vi "run.vi"(8 "error in (no error)":errorcluster, 11 "GenericStimulator in":refnum<class "GenericStimulator.lvclass">) -> (0 "error out":errorcluster, 3 "GenericStimulator out":refnum<class "GenericStimulator.lvclass">)   [LabVIEW 2010, in "GenericStimulator.lvclass"]
uses:
  GenericStimulator.lvclass
panel:
  # "Functionality not available..."
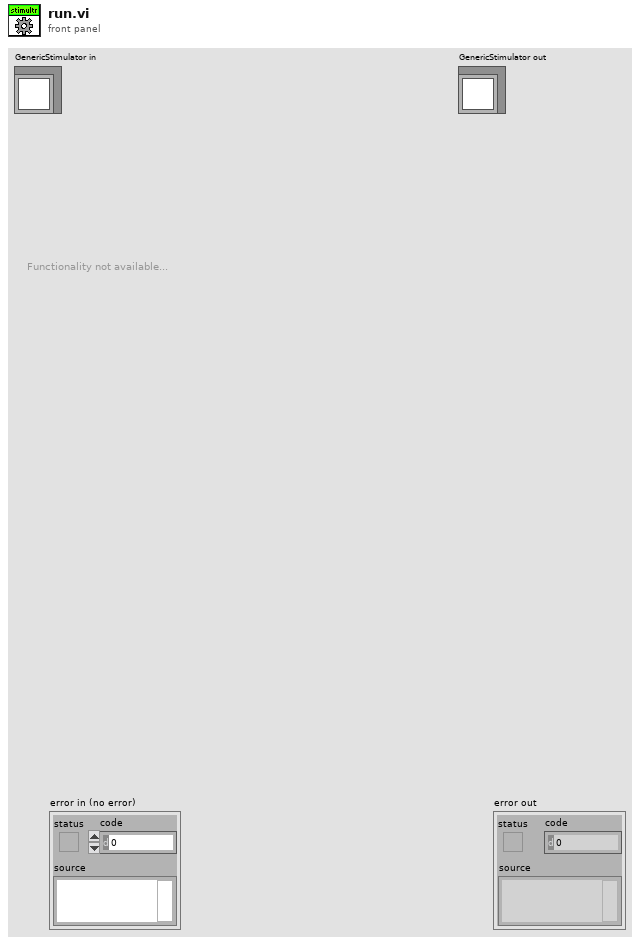
[diagram p1: front panel]
types:
  T1 = typedef "main_trigger_enum.ctl" = enum16{"NULL", "initialise", "terminate", "start", "stop", "change objective", "change experimentController", "change imagingMode", "save notebook", "started saving", "finished saving", "expCtr ready", "expCtr missing", "imgMd ready", "imgMd missing", "scanHd ready", "scanHd missing", "DAQ ready", "DAQ missing", "imgAsm ready", "imgAsm missing", "dataColl ready", "dataColl missing", "display ready", "display missing", "analysr ready", "analysr missing", "instrmnt ready", "instrmnt missing", "stimltr ready", "stimltr missing", "stage ready", "stage missing"}
  T2 = typedef "GenericToplevelComponent.lvclass/common_trigger_enum.ctl" = enum16{"NULL", "initialise", "terminate", "fetch command", "fetch data", "attach observer", "register as observer", "detach observer", "acknowledge", "start", "stop", "sweep started", "sweep finished", "experiment started", "experiment stopped"}
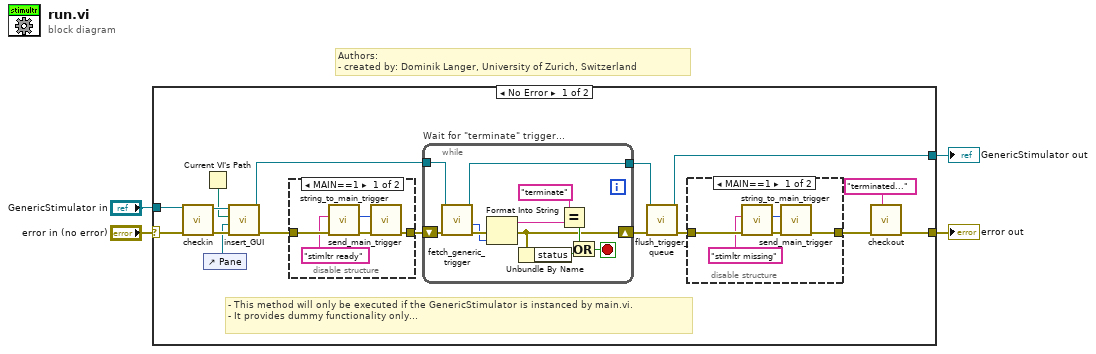
[diagram p0: block diagram]
diagram:
  # "Authors: \n- created by: Dominik Langer, University of Zurich, Switzerland"
  n1 = case shown="No Error" "error in (no error)" {
    selector: "error in (no error)" -> [w20 w45]
    tunnel: [w19 w45] -> w3
    tunnel: [w5 w44] -> w1
    tunnel: "GenericStimulator in" -> [w18 w44]
    frame No Error {
      # "- This method will only be executed if the GenericStimulator is instanced by main.vi.\n- It provides dummy functionality only..."
      n2 = call-dynamic "checkin.vi"("error in (no error)"=w20, "GenericStimulator in"=w18) -> ("error out"=w15:errorcluster, "GenericStimulator out"=w14:refnum<class "GenericStimulator.lvclass">)  [unwired: 8 in]
      n3 = Current VI's Path() -> (path=w13:path)
      n4 = control-ref of="Pane"() -> (w12:refnum<vi>)
      n5 = call-dynamic "insert_GUI.vi"("error in (no error)"=w15, "Pane"=w12, "VI path"=w13, "GenericComponent in"=w14) -> ("error out"=w11:errorcluster, "GenericComponent out"=w6:refnum<class "GenericStimulator.lvclass">)  [unwired: 6 in]
      n6 = disable-structure shown="MAIN==1" {
        disable-tunnel: w11 -> [w30 w32]
        disable-tunnel: [w31 w32] -> w16
        frame condition #0 (active) {
          n7 = call "string_to_main_trigger.vi"("error in (no error)"=w30, "trigger string"="stimltr ready") -> ("error out"=w29:errorcluster, "main trigger"=w28:T1)  [unwired: 8 in]
          n8 = call "send_main_trigger.vi"("error in (no error)"=w29, "trigger"=w28) -> ("error out"=w31:errorcluster)  [unwired: 9 in]
        }
        frame condition #1 {
        }
      }
      n9 = while "Wait for \"terminate\" trigger..." {
        shift-right: [w36] -> w8
        shift-left: w16 -> [w43]
        tunnel: w6 -> [w42]
        tunnel: [w41] -> w9
        stop <- w38 stop-if-true
        n10 = call-dynamic "fetch_generic_trigger.vi"("error in (no error)"=w43, "GenericToplevelComponent in"=w42) -> ("error out"=w37:errorcluster, "common trigger"=w35:T2, "GenericToplevelComponent out"=w41:refnum<class "GenericStimulator.lvclass">)  [unwired: 3 in, 4 out]
        n11 = Format Into String(error in=w37, w35) -> (resulting string=w34:string, error out=w36:errorcluster)  [unwired: 2 in]
        n12 = Unbundle By Name(w36) -> ("status"=w40:bool)
        n13 = Equal?(x="terminate", y=w34) -> (x = y?=w39:bool)
        n14 = Or(x=w39, y=w40) -> (x .or. y?=w38:bool)
      }
      n15 = call-dynamic "flush_trigger_queue.vi"("error in (no error)"=w8, "GenericToplevelComponent in"=w9) -> ("error out"=w7:errorcluster, "GenericToplevelComponent out"=w5:refnum<class "GenericStimulator.lvclass">)  [unwired: 8 in]
      n16 = disable-structure shown="MAIN==1" {
        disable-tunnel: [w25 w26] -> w17
        disable-tunnel: w7 -> [w24 w26]
        frame condition #0 (active) {
          n17 = call "string_to_main_trigger.vi"("error in (no error)"=w24, "trigger string"="stimltr missing") -> ("error out"=w23:errorcluster, "main trigger"=w21:T1)  [unwired: 8 in]
          n18 = call "send_main_trigger.vi"("error in (no error)"=w23, "trigger"=w21) -> ("error out"=w25:errorcluster)  [unwired: 9 in]
        }
        frame condition #1 {
        }
      }
      n19 = call "checkout.vi"("locked by?"="terminated...", "error in (no error)"=w17) -> ("error out"=w19:errorcluster)  [unwired: 8 in, 1 out]
    }
    frame Error {
    }
  }
  "error out" <- w3
  "GenericStimulator out" <- w1
